vi "Configure Math.vi"(7 "Function (0: CH1 + CH2)":i32(ring) items=["CH1 + CH2", "CH1 - CH2", "CH2 - CH1", "CH1 x CH2", "CH3 + CH4", "CH3 - CH4", "CH4 - CH3", "CH3 x CH4", "FFT"], 8 "error in (no error)":errorcluster, 9 "FFT Window (0: Hanning)":i32(ring) items=["Hanning", "Flattop", "Rectangular"], 10 "FFT Channel (1: Channel 1)":i32(ring)=1 items=["Channel 1"=1, "Channel 2"=2, "Channel 3"=3, "Channel 4"=4], 11 "VISA resource name":refnum<visa-resource-name>) -> (0 "error out":errorcluster, 3 "VISA resource out":refnum<visa-resource-name>)   [LabVIEW 2017, in "Tektronix TDS 200 1000 2000 Series.lvlib"]
doc: "Sets the math function to add, subtract, or FFT, and sets FFT properties.\n\n<B>Note(s):</B>\n(1) FFT is only supported for TDS200, TDS 1000/B/C, TDS2000/B/C, and TPS Series.\n(2) For TBS1000B-EDU and TBS1000B series FFT support, please use <B>Configure FFT</B> VI, because FFT button is separated from Math button."
uses:
  Tektronix TDS 200 1000 2000 Series.lvlib
panel:
  # "FFT Settings"
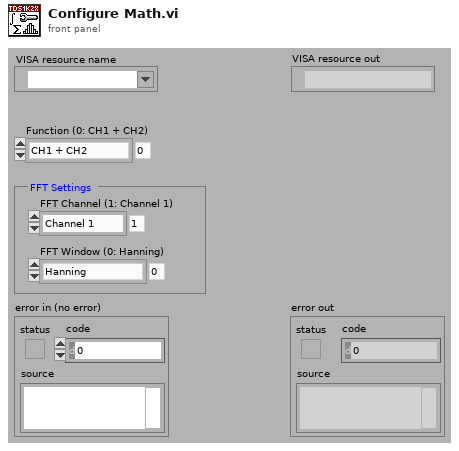
[diagram p1: front panel]
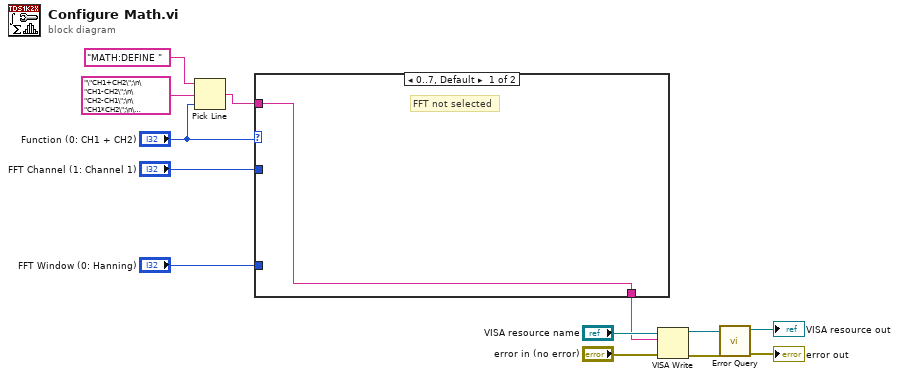
[diagram p0: block diagram]
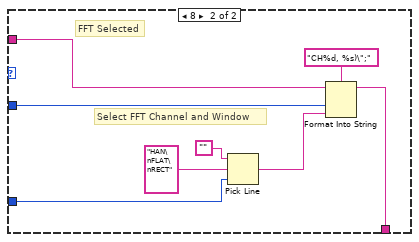
[diagram p2: hidden frame]
diagram:
  n1 = Pick Line(string ("")="MATH:DEFINE ", multi-line string="\"CH1+CH2\";\n\"CH1-CH2\";\n\"CH2-CH1\";\n\"CH1*CH2\";\n\"CH3+CH4\";\n\"CH3-CH4\";\n\"CH4-CH3\";\n\"CH3*CH4\";\n\"FFT (", line index="Function (0: CH1 + CH2)") -> (output string=w10:string)
  n2 = case shown="0..7, Default" "Function (0: CH1 + CH2)" {
    tunnel: w10 -> [w14 w21]
    tunnel: [w14 w17] -> w3
    tunnel: "FFT Channel (1: Channel 1)" -> [_ w16]
    tunnel: "FFT Window (0: Hanning)" -> [_ w15]
    frame 0..7, Default {
      # "FFT not selected"
    }
    frame 8 {
      # "Select FFT Channel and Window"
      # "FFT Selected"
      n3 = Pick Line(string ("")="", multi-line string="HAN\nFLAT\nRECT", line index=w15) -> (output string=w18:string)
      n4 = Format Into String(format string="CH%d, %s)\";", initial string=w21, w16, w18) -> (resulting string=w17:string)  [unwired: 1 in, 1 out]
    }
  }
  n5 = VISA Write(VISA resource name="VISA resource name", write buffer=w3, error in (no error)="error in (no error)") -> (VISA resource name out=w6:refnum<visa-resource-name>, error out=w7:errorcluster)  [unwired: 1 out]
  n6 = call "Error Query.vi"("error in (no error)"=w7, "VISA resource name"=w6) -> ("error out"=→"error out":errorcluster, "VISA resource name out"=→"VISA resource out":refnum<visa-resource-name>)  [unwired: 8 out]
